vi "HOST.vi"() -> ()   [LabVIEW 2018]
uses:
  <vilib>/userdefined/High Color/nirio_resource_hc.ctl
  <vilib>/Analysis/baseanly.llb/Mean (DBL).vi
  <vilib>/FPGAPlugInAG/PXI-7841R/niLvFpga_Open_PXI-7841R.vi
  <vilib>/rvi/interface/common/dynamic/niFpgaDynamicAddResources.vi
  <vilib>/FPGAPlugInAG/Dynamic/niLvFpga_Reset_Dynamic.vi
  <vilib>/FPGAPlugInAG/Dynamic/niLvFpga_Run_Dynamic.vi
  <vilib>/Utility/error.llb/Error Cluster From Error Code.vi
  <vilib>/rvi/errors/niLvFpgaAdjustHostInterfaceError.vi
  <vilib>/FPGAPlugInAG/Dynamic/niLvFpga_Close_Dynamic.vi
  <vilib>/rvi/interface/nirviOpenFPGA/nirviOpenFPGA.xnode
  FPGA Bitfiles/TD_FPGATarget_Target_d-GQJtrYy3M.lvbitx
  <vilib>/rvi/interface/nirviMethod/nirviMethod.xnode
  <vilib>/rvi/interface/nirviReadWriteControl/nirviReadWriteControl.xnode
  <vilib>/rvi/interface/nirviCloseFPGA/nirviCloseFPGA.xnode
  NiFpgaLv.dll
  <vilib>/rvi/interface/Simulation/niFpgaSimulationCallBeginRW.vi
  <vilib>/Analysis/NI_AALBase.lvlib
panel:
  out "VD4_Vcc, В":dbl=1.85440673828125 format="%_4g"
  out "VD4_Vf, В":dbl=0.652301025390625 format="%_4g"
  out "VD4_Vr, В":dbl=1.202105712890625 format="%_4g"
  in  "R4, Ом":dbl=2404.0
  out "VD4_If, мА":dbl=0.5000439737481801 format="%_4g"
  out "VD3_Vcc, В":dbl=1.8546173095703125 format="%_4g"
  out "VD3_Vf, В":dbl=0.6537872314453125 format="%_4g"
  out "VD3_Vr, В":dbl=1.200830078125 format="%_4g"
  in  "R3, Ом":dbl=2401.0
  out "VD3_If, мА":dbl=0.5001374752707206 format="%_4g"
  out "VD2_Vcc, В":dbl=1.8518096923828125 format="%_4g"
  out "VD2_Vf, В":dbl=0.652569580078125 format="%_4g"
  out "VD2_Vr, В":dbl=1.1992401123046874 format="%_4g"
  in  "R2, Ом":dbl=2398.0
  out "VD2_If, мА":dbl=0.5001001302354826 format="%_4g"
  in  "R1, Ом":dbl=2402.0
  out "VD1_Vf, В":dbl=0.6525970458984375 format="%_4g"
  in  "1000?":u16=100
  out "VD1_If, мА":dbl=0.5001134816851843 format="%_4g"
  out "VD1_Vr, В":dbl=1.2012725830078126 format="%_4g"
  out "VD1_Vcc, В":dbl=1.85386962890625 format="%_4g"
  in  "VD4":dbl=1.8559999999999997 format="%_4g"
  in  "VD3":dbl=1.8569999999999995 format="%_4g"
  in  "VD2":dbl=1.8520000000000163 format="%_4g"
  in  "7841":T1="PXI1Slot2"
  in  "VD1":dbl=1.853680000000033 format="%_4g"
  in  "Стоп":bool
  # "Собака-пёс"
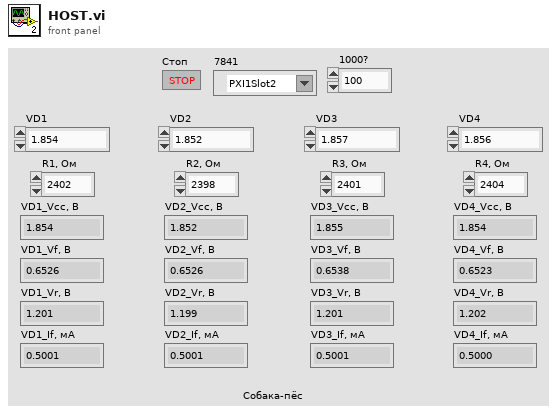
[diagram p1: front panel]
types:
  T1 = typedef "nirio_resource_hc.ctl" = tag
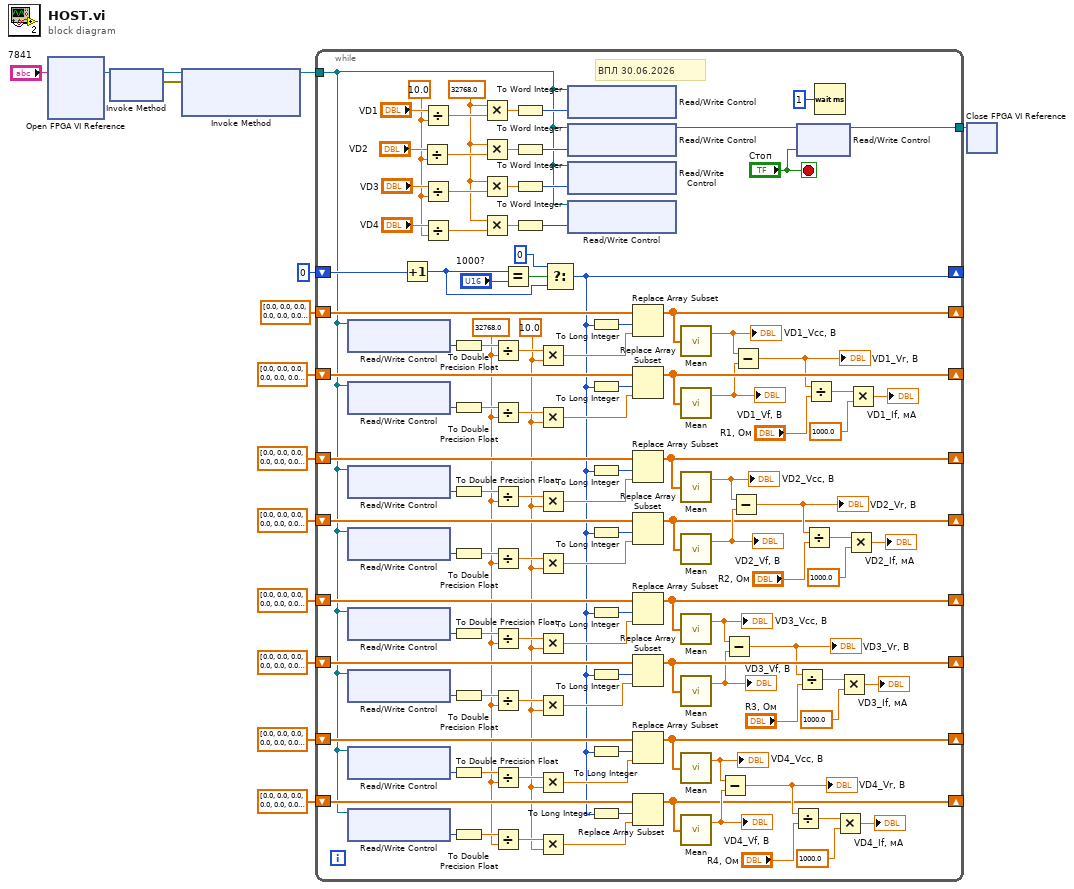
[diagram p0: block diagram]
diagram:
  n1 = xnode "Open FPGA VI Reference"("resource name"="7841") -> ("FPGA VI Reference Out"=w13:refnum<k20>)  [unwired: 1 in, 1 out]
  n2 = xnode "Invoke Method"("FPGA VI Reference In"=w13) -> ("FPGA VI Reference Out"=w15:refnum<k20>, "error out"=w14:errorcluster)  [unwired: 1 in]
  n3 = xnode "Invoke Method"("FPGA VI Reference In"=w15, "error in"=w14) -> ("FPGA VI Reference Out"=w12:refnum<k20>)  [unwired: 1 in, 1 out]
  n4 = while {
    tunnel: w12 -> [w19]
    shift-right: [w16] -> _
    shift-left: u16 0 -> [w107]
    shift-right: [w99] -> _
    shift-left: dbl[] [0.0, 0.0, 0.0, 0.0, 0.0, 0.0, 0.0, 0.0, 0.0, 0.0, 0.0, 0.0, 0.0, 0.0, 0.0, 0.0, 0.0, 0.0, 0.0, 0.0, 0.0, 0.0, 0.0, 0.0, 0.0, 0.0, 0.0, 0.0, 0.0, 0.0, 0.0, 0.0, 0.0, 0.0, 0.0, 0.0, 0.0, 0.0, 0.0, 0.0, 0.0, 0.0, 0.0, 0.0, 0.0, 0.0, 0.0, 0.0, 0.0, 0.0, 0.0, 0.0, 0.0, 0.0, 0.0, 0.0, 0.0, 0.0, 0.0, 0.0, 0.0, 0.0, 0.0, 0.0, 0.0, 0.0, 0.0, 0.0, 0.0, 0.0, 0.0, 0.0, 0.0, 0.0, 0.0, 0.0, 0.0, 0.0, 0.0, 0.0, 0.0, 0.0, 0.0, 0.0, 0.0, 0.0, 0.0, 0.0, 0.0, 0.0, 0.0, 0.0, 0.0, 0.0, 0.0, 0.0, 0.0, 0.0, 0.0, 0.0] ("VD1_Vcc_values") -> [w102]
    shift-right: [w98] -> _
    shift-left: dbl[] [0.0, 0.0, 0.0, 0.0, 0.0, 0.0, 0.0, 0.0, 0.0, 0.0, 0.0, 0.0, 0.0, 0.0, 0.0, 0.0, 0.0, 0.0, 0.0, 0.0, 0.0, 0.0, 0.0, 0.0, 0.0, 0.0, 0.0, 0.0, 0.0, 0.0, 0.0, 0.0, 0.0, 0.0, 0.0, 0.0, 0.0, 0.0, 0.0, 0.0, 0.0, 0.0, 0.0, 0.0, 0.0, 0.0, 0.0, 0.0, 0.0, 0.0, 0.0, 0.0, 0.0, 0.0, 0.0, 0.0, 0.0, 0.0, 0.0, 0.0, 0.0, 0.0, 0.0, 0.0, 0.0, 0.0, 0.0, 0.0, 0.0, 0.0, 0.0, 0.0, 0.0, 0.0, 0.0, 0.0, 0.0, 0.0, 0.0, 0.0, 0.0, 0.0, 0.0, 0.0, 0.0, 0.0, 0.0, 0.0, 0.0, 0.0, 0.0, 0.0, 0.0, 0.0, 0.0, 0.0, 0.0, 0.0, 0.0, 0.0] ("VD1_Vcc_values") -> [w95]
    tunnel: [w83] -> w7
    shift-right: [w68] -> _
    shift-left: dbl[] [0.0, 0.0, 0.0, 0.0, 0.0, 0.0, 0.0, 0.0, 0.0, 0.0, 0.0, 0.0, 0.0, 0.0, 0.0, 0.0, 0.0, 0.0, 0.0, 0.0, 0.0, 0.0, 0.0, 0.0, 0.0, 0.0, 0.0, 0.0, 0.0, 0.0, 0.0, 0.0, 0.0, 0.0, 0.0, 0.0, 0.0, 0.0, 0.0, 0.0, 0.0, 0.0, 0.0, 0.0, 0.0, 0.0, 0.0, 0.0, 0.0, 0.0, 0.0, 0.0, 0.0, 0.0, 0.0, 0.0, 0.0, 0.0, 0.0, 0.0, 0.0, 0.0, 0.0, 0.0, 0.0, 0.0, 0.0, 0.0, 0.0, 0.0, 0.0, 0.0, 0.0, 0.0, 0.0, 0.0, 0.0, 0.0, 0.0, 0.0, 0.0, 0.0, 0.0, 0.0, 0.0, 0.0, 0.0, 0.0, 0.0, 0.0, 0.0, 0.0, 0.0, 0.0, 0.0, 0.0, 0.0, 0.0, 0.0, 0.0] ("VD1_Vcc_values") -> [w65]
    shift-right: [w69] -> _
    shift-left: dbl[] [0.0, 0.0, 0.0, 0.0, 0.0, 0.0, 0.0, 0.0, 0.0, 0.0, 0.0, 0.0, 0.0, 0.0, 0.0, 0.0, 0.0, 0.0, 0.0, 0.0, 0.0, 0.0, 0.0, 0.0, 0.0, 0.0, 0.0, 0.0, 0.0, 0.0, 0.0, 0.0, 0.0, 0.0, 0.0, 0.0, 0.0, 0.0, 0.0, 0.0, 0.0, 0.0, 0.0, 0.0, 0.0, 0.0, 0.0, 0.0, 0.0, 0.0, 0.0, 0.0, 0.0, 0.0, 0.0, 0.0, 0.0, 0.0, 0.0, 0.0, 0.0, 0.0, 0.0, 0.0, 0.0, 0.0, 0.0, 0.0, 0.0, 0.0, 0.0, 0.0, 0.0, 0.0, 0.0, 0.0, 0.0, 0.0, 0.0, 0.0, 0.0, 0.0, 0.0, 0.0, 0.0, 0.0, 0.0, 0.0, 0.0, 0.0, 0.0, 0.0, 0.0, 0.0, 0.0, 0.0, 0.0, 0.0, 0.0, 0.0] ("VD1_Vcc_values") -> [w72]
    shift-right: [w55] -> _
    shift-left: dbl[] [0.0, 0.0, 0.0, 0.0, 0.0, 0.0, 0.0, 0.0, 0.0, 0.0, 0.0, 0.0, 0.0, 0.0, 0.0, 0.0, 0.0, 0.0, 0.0, 0.0, 0.0, 0.0, 0.0, 0.0, 0.0, 0.0, 0.0, 0.0, 0.0, 0.0, 0.0, 0.0, 0.0, 0.0, 0.0, 0.0, 0.0, 0.0, 0.0, 0.0, 0.0, 0.0, 0.0, 0.0, 0.0, 0.0, 0.0, 0.0, 0.0, 0.0, 0.0, 0.0, 0.0, 0.0, 0.0, 0.0, 0.0, 0.0, 0.0, 0.0, 0.0, 0.0, 0.0, 0.0, 0.0, 0.0, 0.0, 0.0, 0.0, 0.0, 0.0, 0.0, 0.0, 0.0, 0.0, 0.0, 0.0, 0.0, 0.0, 0.0, 0.0, 0.0, 0.0, 0.0, 0.0, 0.0, 0.0, 0.0, 0.0, 0.0, 0.0, 0.0, 0.0, 0.0, 0.0, 0.0, 0.0, 0.0, 0.0, 0.0] ("VD1_Vcc_values") -> [w58]
    shift-right: [w54] -> _
    shift-left: dbl[] [0.0, 0.0, 0.0, 0.0, 0.0, 0.0, 0.0, 0.0, 0.0, 0.0, 0.0, 0.0, 0.0, 0.0, 0.0, 0.0, 0.0, 0.0, 0.0, 0.0, 0.0, 0.0, 0.0, 0.0, 0.0, 0.0, 0.0, 0.0, 0.0, 0.0, 0.0, 0.0, 0.0, 0.0, 0.0, 0.0, 0.0, 0.0, 0.0, 0.0, 0.0, 0.0, 0.0, 0.0, 0.0, 0.0, 0.0, 0.0, 0.0, 0.0, 0.0, 0.0, 0.0, 0.0, 0.0, 0.0, 0.0, 0.0, 0.0, 0.0, 0.0, 0.0, 0.0, 0.0, 0.0, 0.0, 0.0, 0.0, 0.0, 0.0, 0.0, 0.0, 0.0, 0.0, 0.0, 0.0, 0.0, 0.0, 0.0, 0.0, 0.0, 0.0, 0.0, 0.0, 0.0, 0.0, 0.0, 0.0, 0.0, 0.0, 0.0, 0.0, 0.0, 0.0, 0.0, 0.0, 0.0, 0.0, 0.0, 0.0] ("VD1_Vcc_values") -> [w51]
    shift-right: [w26] -> _
    shift-left: dbl[] [0.0, 0.0, 0.0, 0.0, 0.0, 0.0, 0.0, 0.0, 0.0, 0.0, 0.0, 0.0, 0.0, 0.0, 0.0, 0.0, 0.0, 0.0, 0.0, 0.0, 0.0, 0.0, 0.0, 0.0, 0.0, 0.0, 0.0, 0.0, 0.0, 0.0, 0.0, 0.0, 0.0, 0.0, 0.0, 0.0, 0.0, 0.0, 0.0, 0.0, 0.0, 0.0, 0.0, 0.0, 0.0, 0.0, 0.0, 0.0, 0.0, 0.0, 0.0, 0.0, 0.0, 0.0, 0.0, 0.0, 0.0, 0.0, 0.0, 0.0, 0.0, 0.0, 0.0, 0.0, 0.0, 0.0, 0.0, 0.0, 0.0, 0.0, 0.0, 0.0, 0.0, 0.0, 0.0, 0.0, 0.0, 0.0, 0.0, 0.0, 0.0, 0.0, 0.0, 0.0, 0.0, 0.0, 0.0, 0.0, 0.0, 0.0, 0.0, 0.0, 0.0, 0.0, 0.0, 0.0, 0.0, 0.0, 0.0, 0.0] ("VD1_Vcc_values") -> [w23]
    shift-right: [w27] -> _
    shift-left: dbl[] [0.0, 0.0, 0.0, 0.0, 0.0, 0.0, 0.0, 0.0, 0.0, 0.0, 0.0, 0.0, 0.0, 0.0, 0.0, 0.0, 0.0, 0.0, 0.0, 0.0, 0.0, 0.0, 0.0, 0.0, 0.0, 0.0, 0.0, 0.0, 0.0, 0.0, 0.0, 0.0, 0.0, 0.0, 0.0, 0.0, 0.0, 0.0, 0.0, 0.0, 0.0, 0.0, 0.0, 0.0, 0.0, 0.0, 0.0, 0.0, 0.0, 0.0, 0.0, 0.0, 0.0, 0.0, 0.0, 0.0, 0.0, 0.0, 0.0, 0.0, 0.0, 0.0, 0.0, 0.0, 0.0, 0.0, 0.0, 0.0, 0.0, 0.0, 0.0, 0.0, 0.0, 0.0, 0.0, 0.0, 0.0, 0.0, 0.0, 0.0, 0.0, 0.0, 0.0, 0.0, 0.0, 0.0, 0.0, 0.0, 0.0, 0.0, 0.0, 0.0, 0.0, 0.0, 0.0, 0.0, 0.0, 0.0, 0.0, 0.0] ("VD1_Vcc_values") -> [w30]
    stop <- "Стоп" stop-if-true
    w17 = 10.0 ("y")
    w18 = 32768.0 ("x")
    w115 = 32768.0 ("x")
    w116 = 10.0 ("y")
    # "ВПЛ 30.06.2026"
    n5 = xnode "Read/Write Control"("FPGA VI Reference In"=w19) -> ("Connector0/AI0"=w110:i16)  [unwired: 1 in, 2 out]
    n6 = xnode "Read/Write Control"("FPGA VI Reference In"=w19) -> ("Connector0/AI1"=w92:i16)  [unwired: 1 in, 2 out]
    n7 = xnode "Read/Write Control"("FPGA VI Reference In"=w19) -> ("Connector0/AI2"=w62:i16)  [unwired: 1 in, 2 out]
    n8 = xnode "Read/Write Control"("FPGA VI Reference In"=w19) -> ("Connector0/AI3"=w75:i16)  [unwired: 1 in, 2 out]
    n9 = xnode "Read/Write Control"("FPGA VI Reference In"=w19) -> ("Connector0/AI4"=w61:i16)  [unwired: 1 in, 2 out]
    n10 = xnode "Read/Write Control"("FPGA VI Reference In"=w19) -> ("Connector0/AI5"=w48:i16)  [unwired: 1 in, 2 out]
    n11 = xnode "Read/Write Control"("FPGA VI Reference In"=w19) -> ("Connector0/AI6"=w20:i16)  [unwired: 1 in, 2 out]
    n12 = xnode "Read/Write Control"("FPGA VI Reference In"=w19) -> ("Connector0/AI7"=w33:i16)  [unwired: 1 in, 2 out]
    n13 = Increment(x=w107) -> (x+1=w103:u16)
    n14 = Divide(x="VD2", y=w116) -> (x/y=w124:dbl)
    n15 = Divide(x="VD1", y=w116) -> (x/y=w127:dbl)
    n16 = Divide(x="VD3", y=w116) -> (x/y=w121:dbl)
    n17 = Divide(x="VD4", y=w116) -> (x/y=w118:dbl)
    n18 = To Double Precision Float(number=w110) -> (double precision float=w109:dbl)
    n19 = To Double Precision Float(number=w92) -> (double precision float=w93:dbl)
    n20 = To Double Precision Float(number=w62) -> (double precision float=w63:dbl)
    n21 = To Double Precision Float(number=w75) -> (double precision float=w74:dbl)
    n22 = To Double Precision Float(number=w61) -> (double precision float=w60:dbl)
    n23 = To Double Precision Float(number=w48) -> (double precision float=w49:dbl)
    n24 = To Double Precision Float(number=w20) -> (double precision float=w21:dbl)
    n25 = To Double Precision Float(number=w33) -> (double precision float=w32:dbl)
    n26 = Multiply(x=w115, y=w127) -> (x*y=w126:dbl)
    n27 = Multiply(x=w115, y=w124) -> (x*y=w125:dbl)
    n28 = Multiply(x=w115, y=w121) -> (x*y=w120:dbl)
    n29 = Multiply(x=w115, y=w118) -> (x*y=w119:dbl)
    n30 = Divide(x=w109, y=w18) -> (x/y=w108:dbl)
    n31 = Divide(x=w93, y=w18) -> (x/y=w94:dbl)
    n32 = Divide(x=w63, y=w18) -> (x/y=w64:dbl)
    n33 = Divide(x=w74, y=w18) -> (x/y=w73:dbl)
    n34 = Divide(x=w60, y=w18) -> (x/y=w59:dbl)
    n35 = Divide(x=w49, y=w18) -> (x/y=w50:dbl)
    n36 = Divide(x=w21, y=w18) -> (x/y=w22:dbl)
    n37 = Divide(x=w32, y=w18) -> (x/y=w31:dbl)
    n38 = Equal?(x=w103, y="1000?") -> (x = y?=w105:bool)
    n39 = To Word Integer(number=w126) -> (16bit integer=w114:i16)
    n40 = To Word Integer(number=w125) -> (16bit integer=w113:i16)
    n41 = To Word Integer(number=w120) -> (16bit integer=w111:i16)
    n42 = To Word Integer(number=w119) -> (16bit integer=w112:i16)
    n43 = Multiply(x=w108, y=w17) -> (x*y=w101:dbl)
    n44 = Multiply(x=w94, y=w17) -> (x*y=w96:dbl)
    n45 = Multiply(x=w64, y=w17) -> (x*y=w66:dbl)
    n46 = Multiply(x=w73, y=w17) -> (x*y=w71:dbl)
    n47 = Multiply(x=w59, y=w17) -> (x*y=w57:dbl)
    n48 = Multiply(x=w50, y=w17) -> (x*y=w52:dbl)
    n49 = Multiply(x=w22, y=w17) -> (x*y=w24:dbl)
    n50 = Multiply(x=w31, y=w17) -> (x*y=w29:dbl)
    n51 = Select(t=u16 0, s=w105, f=w103) -> (s? t:f=w16:u16)
    n52 = xnode "Read/Write Control"("FPGA VI Reference In"=w19, "Connector0/AO0"=w114) -> ()  [unwired: 1 in, 2 out]
    n53 = xnode "Read/Write Control"("FPGA VI Reference In"=w19, "Connector0/AO1"=w113) -> ("FPGA VI Reference Out"=w84:refnum<k20>)  [unwired: 1 in, 1 out]
    n54 = xnode "Read/Write Control"("FPGA VI Reference In"=w19, "Connector0/AO2"=w111) -> ()  [unwired: 1 in, 2 out]
    n55 = xnode "Read/Write Control"("FPGA VI Reference In"=w19, "Connector0/AO3"=w112) -> ()  [unwired: 1 in, 2 out]
    n56 = To Long Integer(number=w16) -> (32bit integer=w100:i32)
    n57 = To Long Integer(number=w16) -> (32bit integer=w97:i32)
    n58 = To Long Integer(number=w16) -> (32bit integer=w67:i32)
    n59 = To Long Integer(number=w16) -> (32bit integer=w70:i32)
    n60 = To Long Integer(number=w16) -> (32bit integer=w56:i32)
    n61 = To Long Integer(number=w16) -> (32bit integer=w53:i32)
    n62 = To Long Integer(number=w16) -> (32bit integer=w25:i32)
    n63 = To Long Integer(number=w16) -> (32bit integer=w28:i32)
    n64 = Replace Array Subset(array=w102, new element=w101, index=w100) -> (w99:dbl[])
    n65 = Replace Array Subset(array=w95, new element=w96, index=w97) -> (w98:dbl[])
    n66 = Replace Array Subset(array=w65, new element=w66, index=w67) -> (w68:dbl[])
    n67 = Replace Array Subset(array=w72, new element=w71, index=w70) -> (w69:dbl[])
    n68 = Replace Array Subset(array=w58, new element=w57, index=w56) -> (w55:dbl[])
    n69 = Replace Array Subset(array=w51, new element=w52, index=w53) -> (w54:dbl[])
    n70 = Replace Array Subset(array=w23, new element=w24, index=w25) -> (w26:dbl[])
    n71 = Replace Array Subset(array=w30, new element=w29, index=w28) -> (w27:dbl[])
    n72 = call-poly <vilib>:"Mean.vi"("X"=w99) -> ("mean"=w91:dbl)  [unwired: 1 out]
    "VD1_Vcc, В" <- w91
    n73 = call-poly <vilib>:"Mean.vi"("X"=w98) -> ("mean"=w90:dbl)  [unwired: 1 out]
    "VD1_Vf, В" <- w90
    n74 = call-poly <vilib>:"Mean.vi"("X"=w68) -> ("mean"=w76:dbl)  [unwired: 1 out]
    "VD2_Vcc, В" <- w76
    n75 = call-poly <vilib>:"Mean.vi"("X"=w69) -> ("mean"=w77:dbl)  [unwired: 1 out]
    "VD2_Vf, В" <- w77
    n76 = call-poly <vilib>:"Mean.vi"("X"=w55) -> ("mean"=w47:dbl)  [unwired: 1 out]
    "VD3_Vcc, В" <- w47
    n77 = call-poly <vilib>:"Mean.vi"("X"=w54) -> ("mean"=w46:dbl)  [unwired: 1 out]
    "VD3_Vf, В" <- w46
    n78 = call-poly <vilib>:"Mean.vi"("X"=w26) -> ("mean"=w34:dbl)  [unwired: 1 out]
    "VD4_Vcc, В" <- w34
    n79 = call-poly <vilib>:"Mean.vi"("X"=w27) -> ("mean"=w35:dbl)  [unwired: 1 out]
    "VD4_Vf, В" <- w35
    n80 = Subtract(x=w34, y=w35) -> (x-y=w36:dbl)
    "VD4_Vr, В" <- w36
    n81 = Subtract(x=w47, y=w46) -> (x-y=w45:dbl)
    "VD3_Vr, В" <- w45
    n82 = Subtract(x=w76, y=w77) -> (x-y=w78:dbl)
    "VD2_Vr, В" <- w78
    n83 = Subtract(x=w91, y=w90) -> (x-y=w89:dbl)
    "VD1_Vr, В" <- w89
    n84 = Divide(x=w36, y="R4, Ом") -> (x/y=w38:dbl)
    n85 = xnode "Read/Write Control"("FPGA VI Reference In"=w84, "Стоп"="Стоп") -> ("FPGA VI Reference Out"=w83:refnum<k20>)  [unwired: 1 in, 1 out]
    n86 = Divide(x=w45, y="R3, Ом") -> (x/y=w43:dbl)
    n87 = Divide(x=w78, y="R2, Ом") -> (x/y=w80:dbl)
    n88 = Divide(x=w89, y="R1, Ом") -> (x/y=w87:dbl)
    n89 = Wait (ms)(milliseconds to wait=u32 1) -> ()  [unwired: 1 out]
    n90 = Multiply(x=w38, y=1000.0) -> (x*y=→"VD4_If, мА":dbl)
    n91 = Multiply(x=w43, y=1000.0) -> (x*y=→"VD3_If, мА":dbl)
    n92 = Multiply(x=w80, y=1000.0) -> (x*y=→"VD2_If, мА":dbl)
    n93 = Multiply(x=w87, y=1000.0) -> (x*y=→"VD1_If, мА":dbl)
  }
  n94 = xnode "Close FPGA VI Reference"("FPGA VI Reference In"=w7) -> ()  [unwired: 1 in, 1 out]
